vi "Read Body.vi"(5 "Upload Path":path=path "", 6 "Max Size (50MB)":u64=52428800, 7 "Uploads as Files? (T)":bool=TRUE, 8 "error in (no error)":errorcluster, 9 "Stream in":refnum<k5>, 11 "Request in":refnum<class "Request.lvclass">) -> (0 "error out":errorcluster, 1 "Stream out":refnum<k5>, 3 "Request out":refnum<class "Request.lvclass">)   [LabVIEW 2020, in "HTTP Utils.lvlib" / "Request.lvclass"]
uses:
  Request.lvclass
  Request.lvclass/Request.ctl
  Multipart Parser/Multipart Parser.lvclass
  lv-stream/stream/Stream/Stream.lvclass
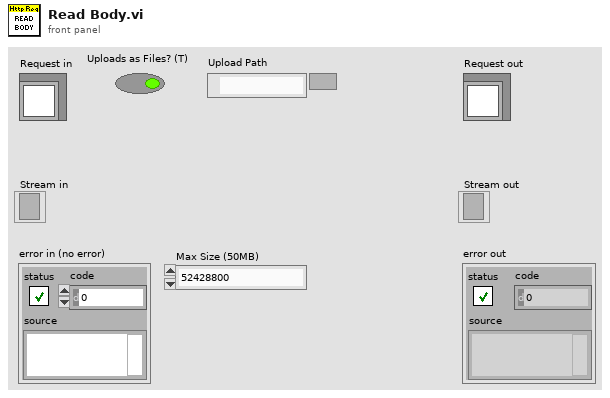
[diagram p1: front panel]
types:
  T1 = typedef "HTTP Utils.lvlib/Request.lvclass/Body Length Type.ctl" = enum16{"Unknown", "Length", "Chunked"}
  T2 = typedef "HTTP Utils.lvlib/Form Type.ctl" = enum16{"None", "UrlEncoded", "Multipart"}
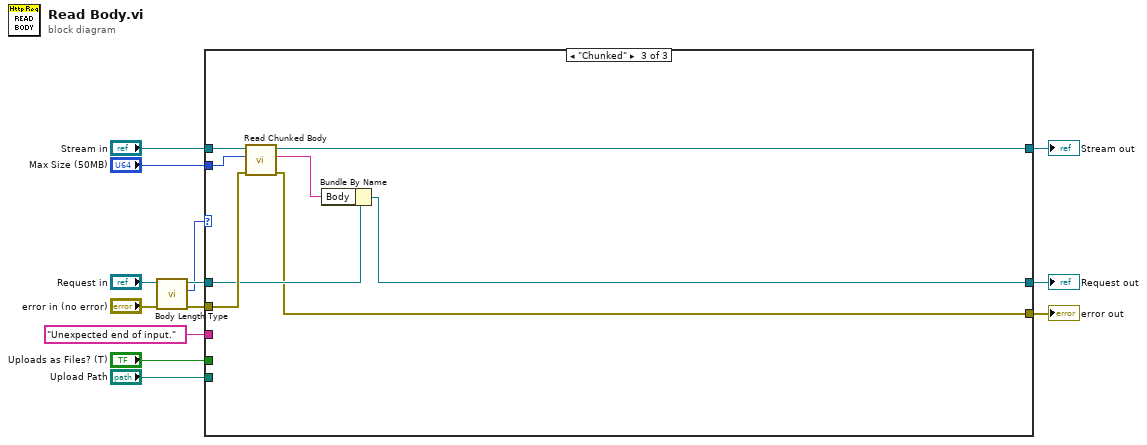
[diagram p0: block diagram]
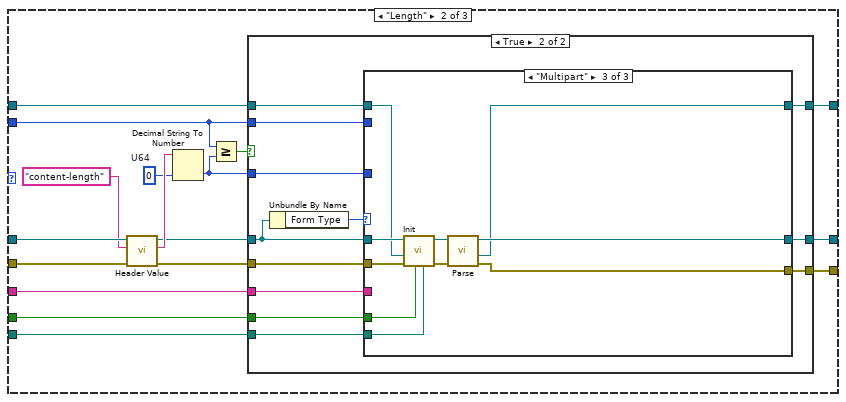
[diagram p3: hidden frame]
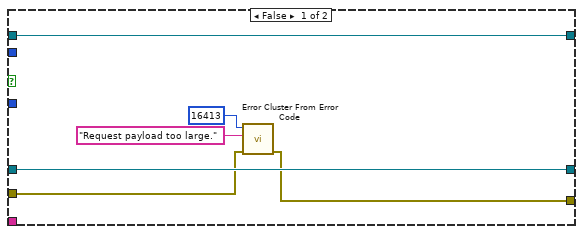
[diagram p4: hidden frame]
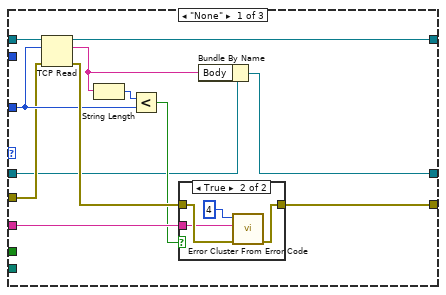
[diagram p5: hidden frame]
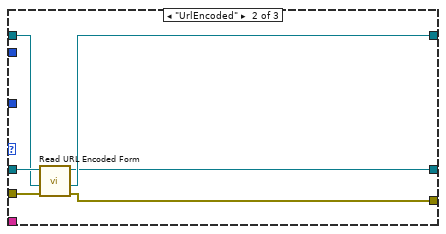
[diagram p7: hidden frame]
diagram:
  n1 = call "Body Length Type.vi"("error in (no error)"="error in (no error)", "Request in"="Request in") -> ("error out"=w10:errorcluster, "Body Length Type"=w9:T1, "Request out"=w11:refnum<class "Request.lvclass">)  [unwired: 7 in]
  n2 = case shown="\"Chunked\"" w9 {
    tunnel: w11 -> [w15 w32 w89]
    tunnel: w10 -> [w14 w31 w91]
    tunnel: "Stream in" -> [w16 w28 w92]
    tunnel: [w16 w27 w90] -> w7
    tunnel: [w15 w25 w86] -> w6
    tunnel: [w14 w24 w87] -> w5
    tunnel: "Unexpected end of input." -> [_ w23 _]
    tunnel: "Max Size (50MB)" -> [_ w19 w85]
    tunnel: "Uploads as Files? (T)" -> [_ w18 _]
    tunnel: "Upload Path" -> [_ w17 _]
    frame "Unknown" {
      # "Requests don't need a length when they have no content.\nPerhaps check for a content-type and only error if there's content-type without length?"
    }
    frame "Length" {
      w21 = u64 0  # U64
      n3 = call "Header Value.vi"("error in (no error)"=w31, "Header"="content-length", "Request in"=w32) -> ("error out"=w33:errorcluster, "Value"=w29:string, "Request out"=w26:refnum<class "Request.lvclass">)  [unwired: 5 in, 1 out]
      n4 = Decimal String To Number(string=w29, default (0L)=w21) -> (number=w22:u64)  [unwired: 1 in, 1 out]
      n5 = Greater Or Equal?(x=w19, y=w22) -> (x >= y?=w20:bool)
      n6 = case shown="True" w20 {
        tunnel: w33 -> [w35 w41]
        tunnel: w28 -> [w39 w51]
        tunnel: [w39 w50] -> w27
        tunnel: w26 -> [w38 w42]
        tunnel: [w38 w49] -> w25
        tunnel: [w34 w48] -> w24
        tunnel: w23 -> [_ w47]
        tunnel: w22 -> [_ w46]
        tunnel: w19 -> [_ w45]
        tunnel: w18 -> [_ w44]
        tunnel: w17 -> [_ w43]
        frame False {
          n7 = call <vilib>:"Error Cluster From Error Code.vi"("error in (no error)"=w35, "error message (\"\")"="Request payload too large." ("error message (\"\")"), "error code (0)"=16413) -> ("error out"=w34:errorcluster)  [unwired: 6 in]
        }
        frame True {
          n8 = Unbundle By Name(w42) -> ("Form Type"=w40:T2)
          n9 = case shown="\"Multipart\"" w40 {
            tunnel: w51 -> [w63 w71 w75]
            tunnel: [w62 w70 w76] -> w50
            tunnel: [w61 w69 w77] -> w49
            tunnel: [w57 w72 w78] -> w48
            tunnel: w47 -> [w56 _ _]
            tunnel: w46 -> [w54 _ _]
            tunnel: w41 -> [w53 w73 w83]
            tunnel: w42 -> [w52 w74 w84]
            tunnel: w45 -> [_ _ _]
            tunnel: w44 -> [_ _ w82]
            tunnel: w43 -> [_ _ w81]
            frame "None" {
              n10 = TCP Read(connection ID=w63, bytes to read=w54, error in (no error)=w53) -> (connection ID out=w62:refnum<k5>, data out=w60:string, error out=w58:errorcluster)  [unwired: 2 in]
              n11 = String Length(string=w60) -> (length=w59:i32)
              n12 = Less?(x=w59, y=w54) -> (x < y?=w55:bool)
              n13 = case shown="True" w55 {
                tunnel: w58 -> [w64 w66]
                tunnel: [w64 w68] -> w57
                tunnel: w56 -> [_ w65]
                frame False {
                }
                frame True {
                  n14 = call <vilib>:"Error Cluster From Error Code.vi"("error in (no error)"=w66, "error message (\"\")"=w65, "error code (0)"=4) -> ("error out"=w68:errorcluster)  [unwired: 6 in]
                }
              }
              n15 = Bundle By Name(cluster=w52, "Body"=w60) -> (w61:refnum<class "Request.lvclass">)
            }
            frame "UrlEncoded" {
              n16 = call "Read URL Encoded Form.vi"("error in (no error)"=w73, "Stream in"=w71, "Request in"=w74) -> ("error out"=w72:errorcluster, "Stream out"=w70:refnum<k5>, "Request out"=w69:refnum<class "Request.lvclass">)  [unwired: 6 in]
            }
            frame "Multipart" {
              n17 = call "Init.vi"("Upload Path"=w81, "Uploads as Files?"=w82, "error in (no error)"=w83, "Stream"=w75, "Request"=w84) -> ("error out"=w79:errorcluster, "Multipart Parser out"=w80:refnum<class "Multipart Parser.lvclass">)  [unwired: 5 in]
              n18 = call "Parse.vi"("error in (no error)"=w79, "Multipart Parser in"=w80) -> ("error out"=w78:errorcluster, "Stream"=w76:refnum<k5>, "Request"=w77:refnum<class "Request.lvclass">)  [unwired: 7 in]
            }
          }
        }
      }
    }
    frame "Chunked" {
      n19 = call "Read Chunked Body.vi"("error in (no error)"=w91, "Max Size (50MB)"=w85, "Stream in"=w92) -> ("error out"=w87:errorcluster, "Body"=w88:string, "Stream out"=w90:refnum<k5>)  [unwired: 6 in]
      n20 = Bundle By Name(cluster=w89, "Body"=w88) -> (w86:refnum<class "Request.lvclass">)
    }
  }
  "error out" <- w5
  "Request out" <- w6
  "Stream out" <- w7
